vi "TomsToolsDocumentationTool_Global_Init.vi"(11 "Object":T1) -> ()   [LabVIEW 2015]
uses:
  <resource>/Framework/Providers/API/mxLvMenuItem.ctl
  <resource>/Framework/Providers/API/ItemRef.ctl
panel:
  out "error out":errorcluster
  in  "error in":errorcluster
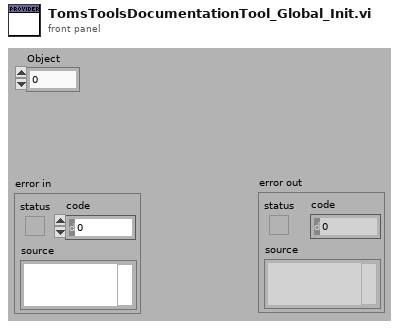
[diagram p1: front panel]
types:
  T1 = typedef "ItemRef.ctl" = u64
  T2 = typedef "mxLvMenuItem.ctl" = cluster{"Menu Name":string, "Description":string, "Icon File Name":path, "Menu Tag":string, "Enabled":bool, "Checked":bool, "Separator":bool, "Batchable":bool, "Weight":i32, "Batch Mode (Ignored if Not Batchable)":enum32{"Show If All Items Support Command", "Show If Any Items Support Command"}, "Menu Location":enum32{"<None>", "Project", "Project / Build Specifications", "Tools", "Tools / Source Control", "Tools / Real-Time Module", "Help"}, "Exclude From Getting Started Window Menu":bool}
  T3 = enum32{"<None>", "Project", "Project / Build Specifications", "Tools", "Tools / Source Control", "Tools / Real-Time Module", "Help"}
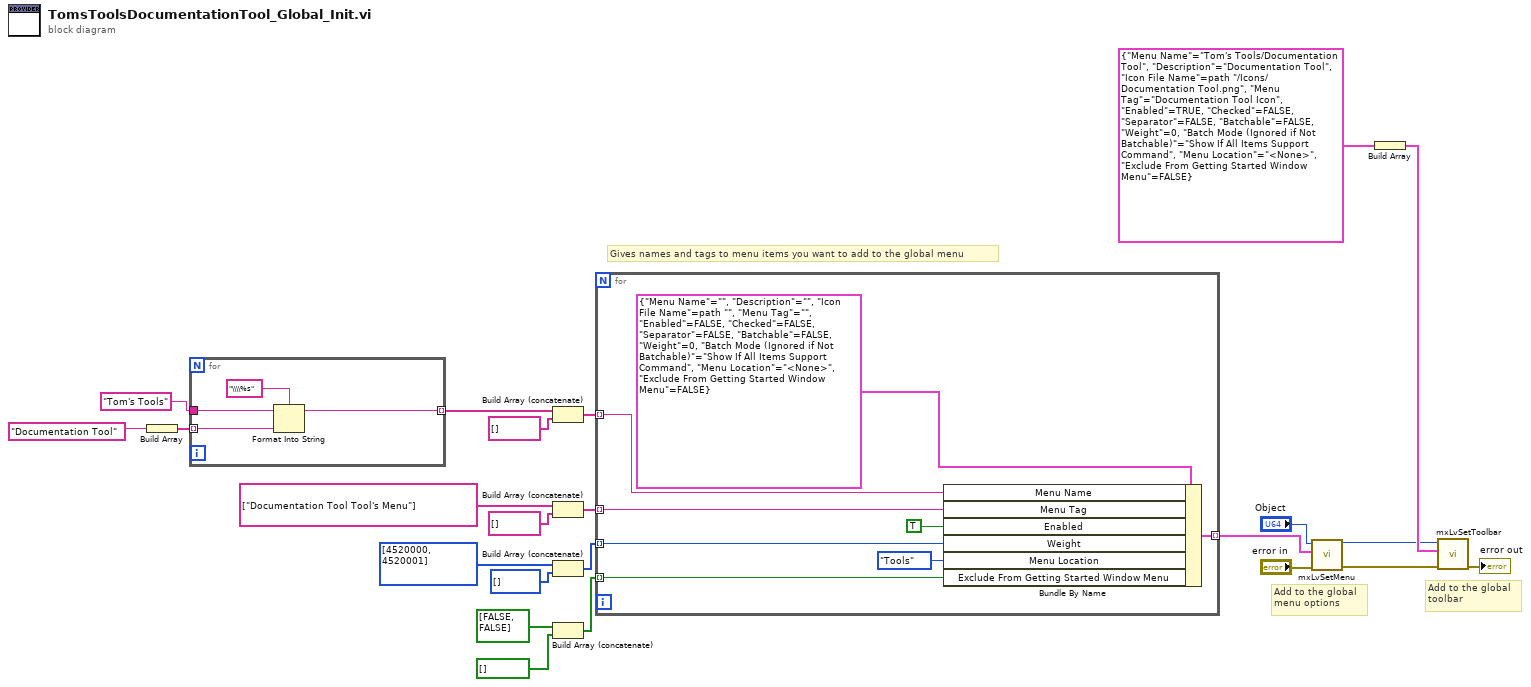
[diagram p0: block diagram]
diagram:
  # "Add to the global\ntoolbar"
  # "Add to the global\nmenu options"
  # "Gives names and tags to menu items you want to add to the global menu"
  n1 = Build Array("Documentation Tool" ("SecondaryProviderExample1")) -> (w17:string[])
  n2 = for {
    tunnel: w17 -> [w24] mode=indexing
    tunnel: "Tom's Tools" ("SecondaryProviderExample1") -> [w27]
    tunnel: [w26] -> w16 mode=indexing
    n3 = Format Into String(format string="\\\\%s", initial string=w27, w24) -> (resulting string=w26:string)  [unwired: 1 in, 1 out]
  }
  n4 = Build Array (concatenate)(w16, string[] [] ("array")) -> (w15:string[])
  n5 = Build Array (concatenate)(string[] ["Documentation Tool Tool's Menu"] ("menu tag"), string[] [] ("array")) -> (w14:string[])
  n6 = Build Array (concatenate)(i32[] [4520000, 4520001] ("menu weight"), i32[] [] ("array")) -> (w13:i32[])
  n7 = Build Array (concatenate)(bool[] [FALSE, FALSE] ("exclude from GSW"), bool[] [] ("array")) -> (w12:bool[])
  n8 = for {
    tunnel: [w35] -> w20 mode=indexing
    tunnel: w13 -> [w34] mode=indexing
    tunnel: w14 -> [w33] mode=indexing
    tunnel: w15 -> [w31] mode=indexing
    tunnel: w12 -> [w32] mode=indexing
    n9 = Bundle By Name(cluster=T2 {"Menu Name"="", "Description"="", "Icon File Name"=path "", "Menu Tag"="", "Enabled"=FALSE, "Checked"=FALSE, "Separator"=FALSE, "Batchable"=FALSE, "Weight"=0, "Batch Mode (Ignored if Not Batchable)"=enum."Show If All Items Support Command", "Menu Location"=enum."<None>", "Exclude From Getting Started Window Menu"=FALSE} ("Menu Item"), "Menu Name"=w31, "Menu Tag"=w33, "Enabled"=TRUE ("Checked"), "Weight"=w34, "Menu Location"=T3."Tools", "Exclude From Getting Started Window Menu"=w32) -> (w35:T2)
  }
  n10 = call <resource>:"mxLvSetMenu.vi"("error in"="error in", "Menu Items"=w20, "Item"="Object") -> ("error out"=w3:errorcluster, "Item"=w5:T1)  [unwired: 7 out]
  n11 = Build Array(T2 {"Menu Name"="Tom's Tools/Documentation Tool", "Description"="Documentation Tool", "Icon File Name"=path "../Icons/Documentation Tool.png", "Menu Tag"="Documentation Tool Icon", "Enabled"=TRUE, "Checked"=FALSE, "Separator"=FALSE, "Batchable"=FALSE, "Weight"=0, "Batch Mode (Ignored if Not Batchable)"=enum."Show If All Items Support Command", "Menu Location"=enum."<None>", "Exclude From Getting Started Window Menu"=FALSE} ("Menu Item")) -> (w7:T2[])
  n12 = call <resource>:"mxLvSetToolbar.vi"("error in"=w3, "Toolbar Items"=w7, "Item"=w5) -> ("error out"=→"error out":errorcluster)  [unwired: 7 in, 1 out]
